vi "Pre-Reanimate.vi"(6 "Search Path":path[](array[path]), 8 "Error In":errorcluster, 10 "Grave In":refnum<vi>, 11 "VI In":refnum<vi>) -> (0 "Error Out":errorcluster, 2 "Grave Out":refnum<vi>, 3 "VI Out":refnum<vi>)   [LabVIEW 2018, in "Toolkit.lvlib"]
uses:
  Toolkit.lvlib
  Typedefs/Hooks.ctl
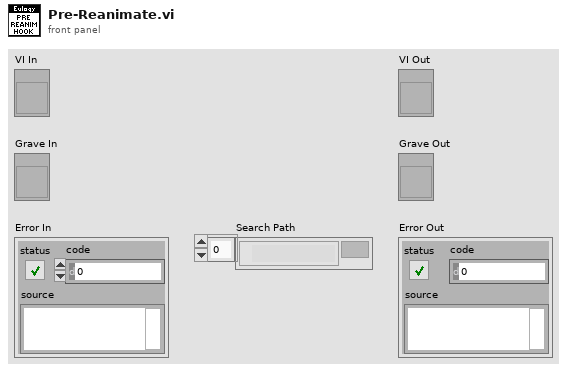
[diagram p1: front panel]
types:
  T1 = typedef "Toolkit.lvlib/Hooks.ctl" = enum16{"Pre-Bury", "Post-Bury", "Pre-Dig", "Post-Dig", "Pre-Reanimate", "Post-Reanimate", "Pre-Smite", "Post-Smite"}
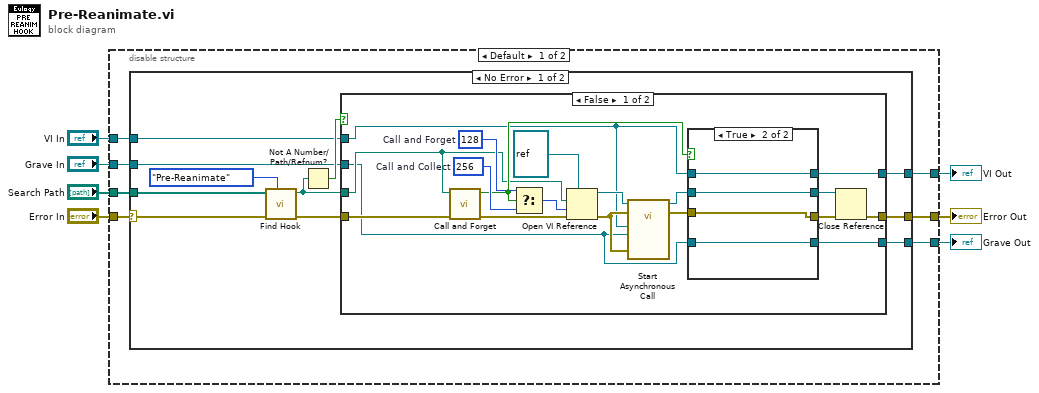
[diagram p0: block diagram]
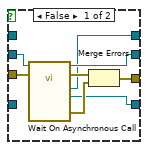
[diagram p2: hidden frame]
diagram:
  n1 = disable-structure "Conditional Disable Structure" shown="Default" {
    disable-tunnel: [w14 w63] -> w7
    disable-tunnel: "Error In" -> [w13 w63]
    disable-tunnel: "Search Path" -> [w12 _]
    disable-tunnel: "Grave In" -> [w11 w64]
    disable-tunnel: [w10 w64] -> w3
    disable-tunnel: "VI In" -> [w9 w65]
    disable-tunnel: [w8 w65] -> w1
    frame condition #0 (active) {
      n2 = case shown="No Error" w13 {
        selector: w13 -> [w23 w62]
        tunnel: [w24 w62] -> w14
        tunnel: w12 -> [w16 _]
        tunnel: w11 -> [w20 w61]
        tunnel: [w19 w61] -> w10
        tunnel: w9 -> [w18 w60]
        tunnel: [w17 w60] -> w8
        frame No Error {
          n3 = call "Find Hook.vi"("Hook"=Hooks."Pre-Reanimate", "Error In"=w23, "Search Path"=w16) -> ("Error Out"=w25:errorcluster, "Hook"=w22:path)  [unwired: 7 in]
          n4 = Not A Number/Path/Refnum?(number/path/refnum=w22) -> (NaN/Path/Refnum?=w21:bool)
          n5 = case shown="False" w21 {
            tunnel: w22 -> [w32 _]
            tunnel: w25 -> [w36 w59]
            tunnel: [w44 w59] -> w24
            tunnel: w20 -> [w28 w58]
            tunnel: [w31 w58] -> w19
            tunnel: w18 -> [w26 w57]
            tunnel: [w27 w57] -> w17
            frame False {
              w38 = 256  # Call and Collect
              w39 = 128  # Call and Forget
              n6 = call "Call and Forget.vi"("Error In"=w36, "Hook"=w32) -> ("Error Out"=w35:errorcluster, "Call and Forget"=w34:bool)  [unwired: 8 in]
              n7 = Select(t=w39, s=w34, f=w38) -> (s? t:f=w37:i32)
              n8 = Open VI Reference(type specifier VI Refnum (for type only)=refnum<vi> refnum, vi path=w32, options=w37, error in (no error)=w35) -> (vi reference=w29:refnum<vi>, error out=w33:errorcluster)  [unwired: 2 in]
              n9 = call-by-ref "Start Asynchronous Call"(reference=w29, error in=w33, "Error In"=w33, "Grave In"=w28, "VI In"=w26) -> (reference out=w43:refnum<vi>, error out=w41:errorcluster)  [unwired: 6 in, 3 out]
              n10 = case shown="True" w34 {
                tunnel: w43 -> [w52 w56]
                tunnel: [w51 w56] -> w42
                tunnel: w41 -> [w50 w55]
                tunnel: [w48 w55] -> w40
                tunnel: w28 -> [_ w54]
                tunnel: [w46 w54] -> w31
                tunnel: [w45 w53] -> w27
                tunnel: w26 -> [_ w53]
                frame False {
                  n11 = call-by-ref "Wait On Asynchronous Call"(reference=w52, error in=w50) -> (reference out=w51:refnum<vi>, error out=w49:errorcluster, "Error Out"=w47:errorcluster, "Grave Out"=w46:refnum<vi>, "VI Out"=w45:refnum<vi>)  [unwired: 9 in]
                  n12 = Merge Errors(w49, w47) -> (w48:errorcluster)
                }
                frame True {
                }
              }
              n13 = Close Reference(reference=w42, error in (no error)=w40) -> (error out=w44:errorcluster)
            }
            frame True {
            }
          }
        }
        frame Error {
        }
      }
    }
    frame condition #1 {
    }
  }
  "Error Out" <- w7
  "Grave Out" <- w3
  "VI Out" <- w1
